vi "ArmSetUpDown.vi"(8 "ArmUpDown":bool) -> ()   [LabVIEW 2020]
doc: "Arm Setter for up down \nInputs:\n--ArmUpDown--Boolean--"
uses:
  ArmGlobal.vi
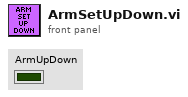
[diagram p1: front panel]
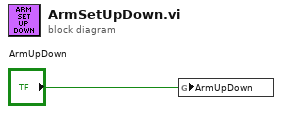
[diagram p0: block diagram]
diagram:
  n1 = global write "ArmGlobal.vi" "ArmUpDown"("ArmUpDown") -> ()
